vi "Merge.vi"(9 "new message":refnum<class "Channel Message.lvclass">, 11 "already enqueued message":refnum<class "Channel Message.lvclass">) -> (1 "merged?":bool, 3 "merged message":refnum<class "Channel Message.lvclass">)   [LabVIEW 2017, in "Channel Message.lvclass"]
doc: "When a message is written into a Messenger channel, the normal behavior is to just add it as the new last element of the channel. However, some applications prefer to consolidate duplicate messages. Override this method to decide whether two messages in the channel should be merged. If they should be merged, output the merged message and True. Otherwise output the unmodified \"already enqueued message\" and False.\n\nThe Messgener only merges the very last message already in the channel with the new message being written. It will not attempt to merge with the rest of the messages in the channel."
uses:
  <vilib>/ChannelSupport/Channel Message/Channel Message.lvclass
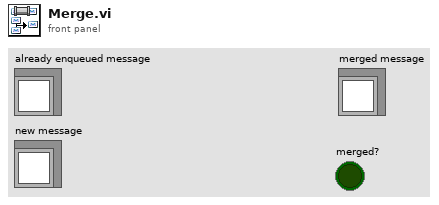
[diagram p1: front panel]
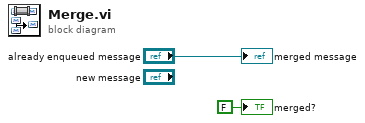
[diagram p0: block diagram]
diagram:
  "merged message" <- "already enqueued message"
  "merged?" <- FALSE ("merged?")
